vi "get_shape.vi"(8 "error in (no error)":errorcluster, 11 "Interface_get_shape in":refnum<class "Interface_get_shape.lvclass">) -> (0 "error out":errorcluster, 2 "out 2":cluster{"n_rows":dbl, "n_cols":dbl}, 3 "Interface_get_shape out":refnum<class "Interface_get_shape.lvclass">)   [LabVIEW 2020, in "Interface_get_shape.lvclass"]
doc: "Shape of the i’th bicluster."
uses:
  Interface_get_shape.lvclass
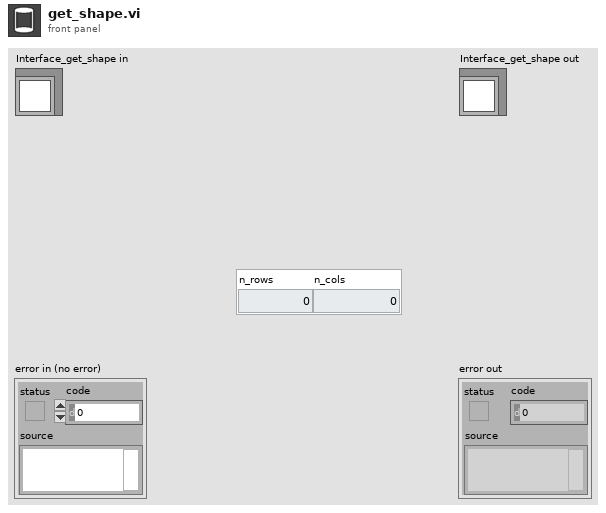
[diagram p1: front panel]
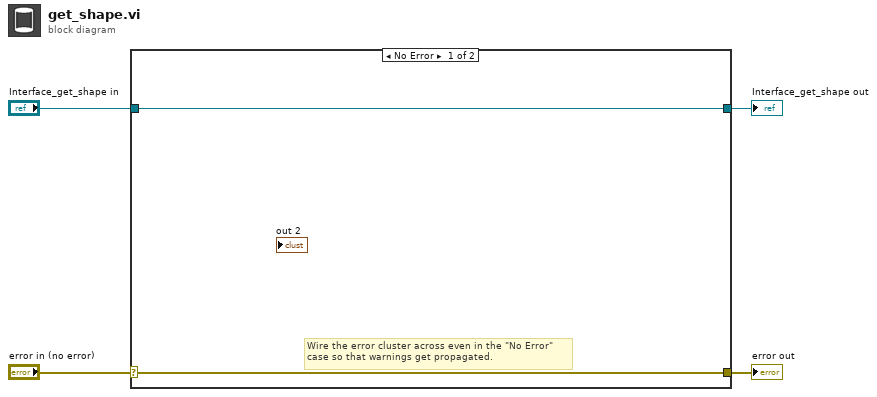
[diagram p0: block diagram]
diagram:
  n1 = case shown="No Error" "error in (no error)" {
    selector: "error in (no error)" -> [w5 w8]
    tunnel: [w5 w8] -> w3
    tunnel: [w6 w7] -> w1
    tunnel: "Interface_get_shape in" -> [w6 w7]
    frame No Error {
      # "Wire the error cluster across even in the \"No Error\"\ncase so that warnings get propagated."
    }
    frame Error {
    }
  }
  "error out" <- w3
  "Interface_get_shape out" <- w1
